vi "Set CurWeek.vi"(8 "error in (no error)":errorcluster, 10 "CurWeek(0)":i32, 11 "Admin_Actor in":refnum<class "Admin_Actor.lvclass">) -> (0 "error out":errorcluster, 3 "Admin_Actor out":refnum<class "Admin_Actor.lvclass">)   [LabVIEW 2015, in "Admin_Actor.lvlib" / "Admin_Actor.lvclass"]
uses:
  Admin_Actor.lvclass
  Admin_Actor.lvclass/Admin_Actor.ctl
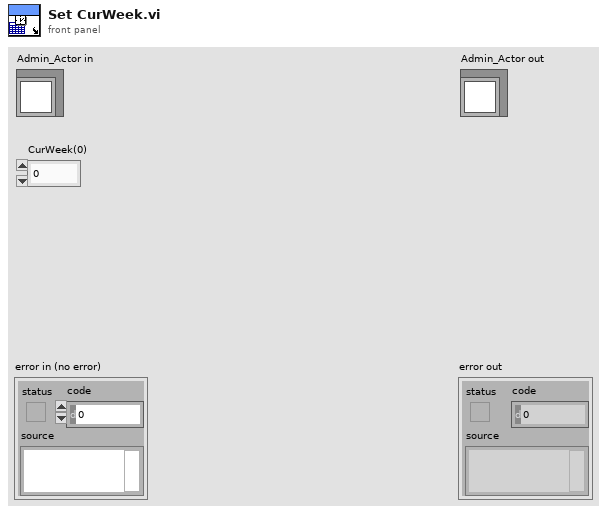
[diagram p1: front panel]
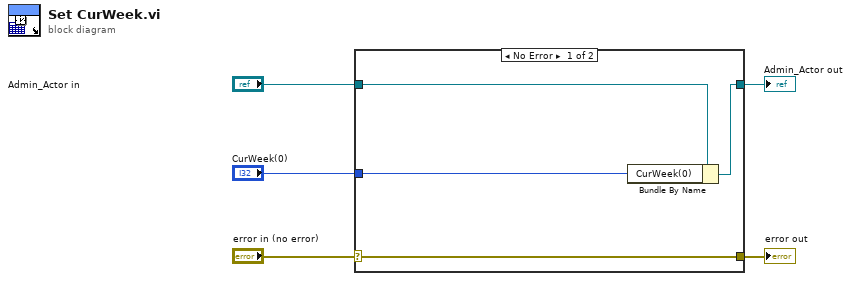
[diagram p0: block diagram]
diagram:
  n1 = case shown="No Error" "error in (no error)" {
    selector: "error in (no error)" -> [w9 w10]
    tunnel: [w9 w10] -> w4
    tunnel: [w7 w11] -> w2
    tunnel: "Admin_Actor in" -> [w8 w11]
    tunnel: "CurWeek(0)" -> [w6 _]
    frame No Error {
      n2 = Bundle By Name(cluster=w8, "CurWeek(0)"=w6) -> (w7:refnum<class "Admin_Actor.lvclass">)
    }
    frame Error {
    }
  }
  "error out" <- w4
  "Admin_Actor out" <- w2
